vi "Voltage to Z-position OLD.vi"(11 "Voltage":dbl) -> (3 "Position":dbl)   [LabVIEW 2012]
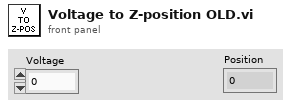
[diagram p1: front panel]
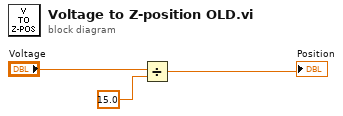
[diagram p0: block diagram]
diagram:
  n1 = Divide(x="Voltage", y=15.0) -> (x/y=→"Position":dbl)
